vi "Extract positional data on selected miniscan.vi"(8 "error in (no error)":errorcluster, 9 "Display State In":T1={"Numeric"=0.0, "Timeline Ref"=refnum, "Waveform Ref"=refnum, "Fill Plots"=FALSE, "Cursor Redraw"=TRUE}, 11 "Data In":T4) -> (0 "error out":errorcluster, 1 "Extracted intensity data at selected mini-scan location":sgl[](graph))   [LabVIEW 2017, in "XGrapher.xctl"]
uses:
  XGrapher.xctl
  Data 1.ctl
  Typedefs/Xctrl-Data array.ctl
  Typedefs/Xcrtl-Data format definition.ctl
  Typedefs/Xctl-XY data type definition.ctl
  Typedefs/Xctrl-ROI type enum.ctl
  State 1.ctl
  Typedefs/Xctrl-Timeline graph ref.ctl
  Typedefs/Xctrl-Waveform graph ref.ctl
  <userlib>/_OpenG.lib/array/array.llb/Index 1D Array Elements (SGL)__ogtk.vi
panel:
  out "Number of cycles":i32
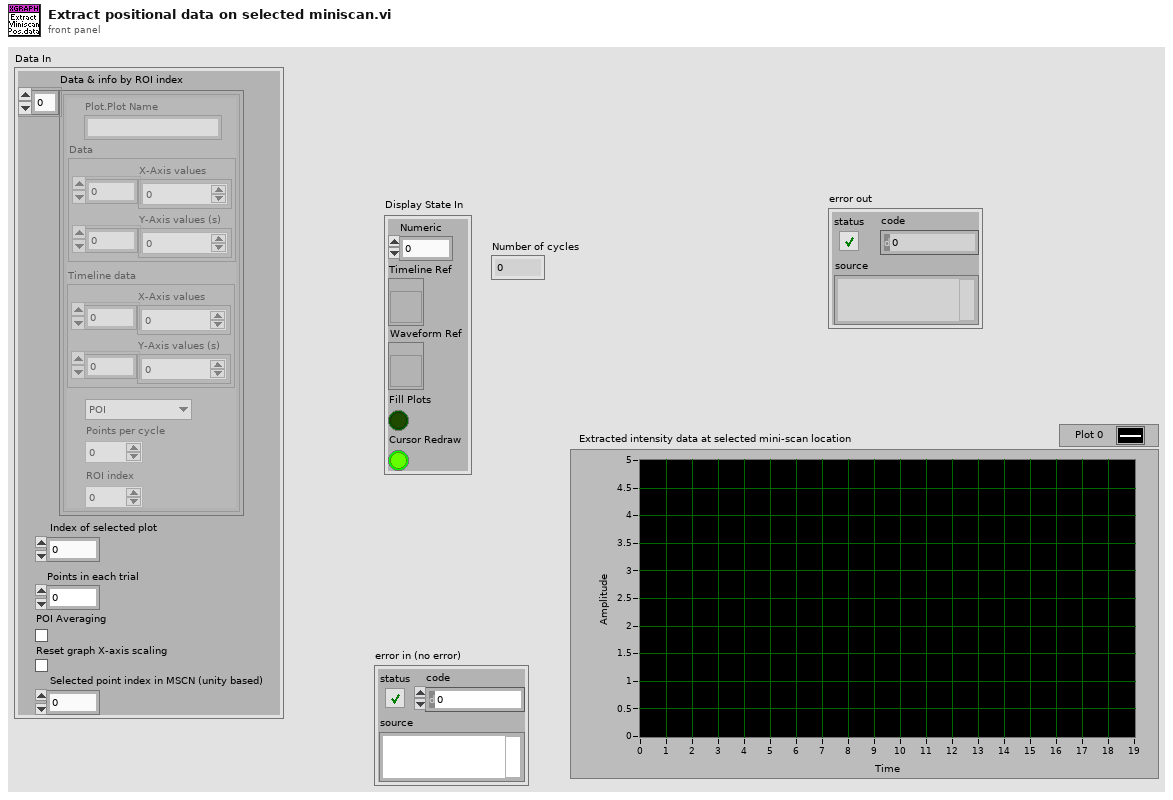
[diagram p1: front panel]
types:
  T1 = typedef "XGrapher.xctl/State 1.ctl" = cluster{"Numeric":dbl, "Timeline Ref":T2, "Waveform Ref":T3, "Fill Plots":bool, "Cursor Redraw":bool}
  T2 = typedef "XGrapher.xctl/Xctrl-Timeline graph ref.ctl" = refnum<vi>
  T3 = typedef "XGrapher.xctl/Xctrl-Waveform graph ref.ctl" = refnum<vi>
  T4 = typedef "XGrapher.xctl/Data 1.ctl" = cluster{"Data & info by ROI index":T5, "Index of selected plot":u16, "Points in each trial":i32, "POI Averaging":bool, "Reset graph X-axis scaling":bool, "Selected point index in MSCN (unity based)":u16}
  T5 = typedef "Xctrl-Data array.ctl" = T6[]
  T6 = typedef "XGrapher.xctl/Xcrtl-Data format definition.ctl" = cluster{"Plot.Plot Name":string, "Data":T7, "Timeline data":T7, "Type":T8, "Points per cycle":u16, "ROI index":u16}
  T7 = typedef "XGrapher.xctl/Xctl-XY data type definition.ctl" = cluster{"X-Axis values":sgl[], "Y-Axis values (s)":sgl[]}
  T8 = typedef "Xctrl-ROI type enum.ctl" = enum16{"POI", "Mini-scan", "Group"}
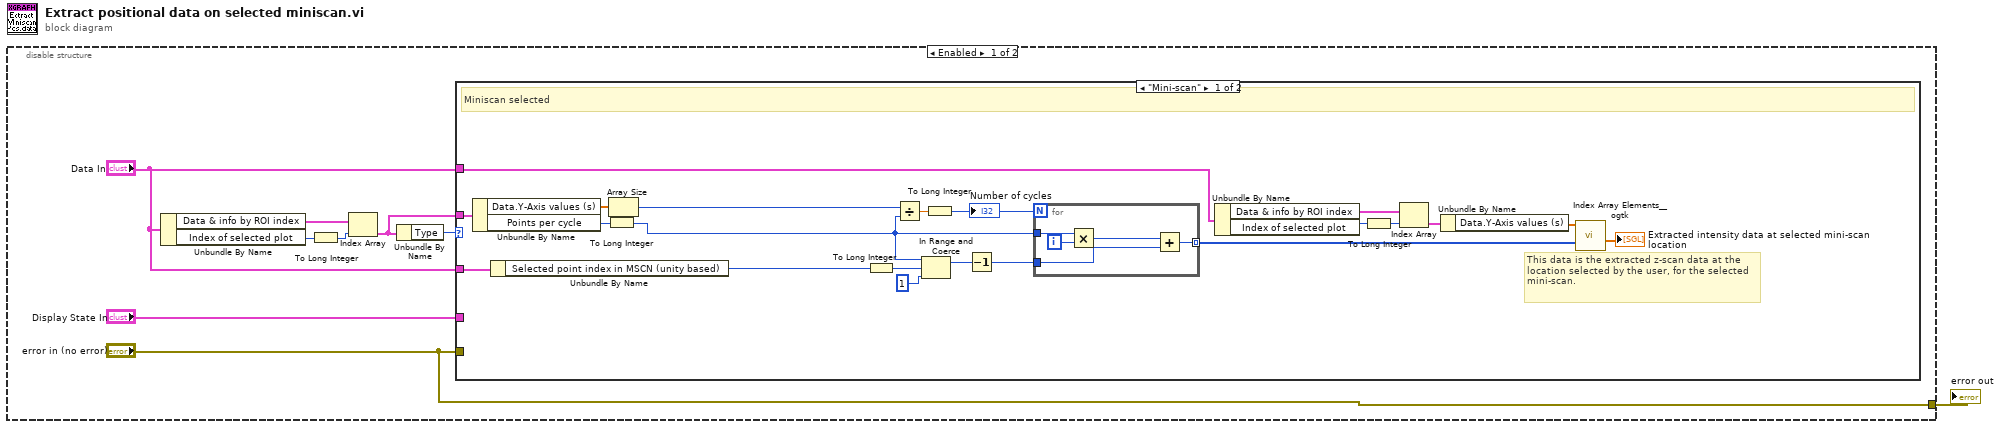
[diagram p0: block diagram]
diagram:
  n1 = disable-structure shown="Enabled" {
    disable-tunnel: ["error in (no error)" _] -> w1
    frame Enabled {
      n2 = Unbundle By Name("Data In") -> ("Data & info by ROI index"=w7:T5, "Index of selected plot"=w8:u16)
      n3 = To Long Integer(number=w8) -> (32bit integer=w6:i32)
      n4 = Index Array(array=w7, index=w6) -> (element=w4:T6)
      n5 = Unbundle By Name(w4) -> ("Type"=w5:T8)
      n6 = case shown="\"Mini-scan\"" w5 {
        tunnel: "Data In" -> [w18 _]
        tunnel: "Display State In" -> [_ _]
        tunnel: "error in (no error)" -> [_ _]
        tunnel: w4 -> [w19 _]
        tunnel: "Data In" -> [w16 _]
        frame "Mini-scan" {
          # "This data is the extracted z-scan data at the location selected by the user, for the selected mini-scan."
          # "Miniscan selected"
          n7 = Unbundle By Name(w19) -> ("Data.Y-Axis values (s)"=w24:sgl[], "Points per cycle"=w15:u16)
          n8 = Unbundle By Name(w16) -> ("Selected point index in MSCN (unity based)"=w17:u16)
          n9 = To Long Integer(number=w15) -> (32bit integer=w13:i32)
          n10 = Array Size(array=w24) -> (size(s)=w27:i32)
          n11 = To Long Integer(number=w17) -> (32bit integer=w10:i32)
          n12 = Divide(x=w27, y=w13) -> (x/y=w26:dbl)
          n13 = In Range and Coerce(upper limit=w13, x=w10, lower limit=1) -> (coerced(x)=w12:i32)  [unwired: 1 out]
          n14 = To Long Integer(number=w26) -> (32bit integer=w25:i32)
          "Number of cycles" <- w25
          n15 = Decrement(x=w12) -> (x-1=w11:i32)
          n16 = for {
            N: w25 -> [_]
            tunnel: [w32] -> w23 mode=indexing
            tunnel: w13 -> [w34]
            tunnel: w11 -> [w31]
            i -> [w35]
            n17 = Multiply(x=w34, y=w35) -> (x*y=w33:i32)
            n18 = Add(x=w33, y=w31) -> (x+y=w32:i32)
          }
          n19 = Unbundle By Name(w18) -> ("Data & info by ROI index"=w29:T5, "Index of selected plot"=w30:u16)
          n20 = To Long Integer(number=w30) -> (32bit integer=w28:i32)
          n21 = Index Array(array=w29, index=w28) -> (element=w22:T6)
          n22 = Unbundle By Name(w22) -> ("Data.Y-Axis values (s)"=w21:sgl[])
          n23 = call-poly <userlib>:"Index Array Elements__ogtk.vi"("indices"=w23, "array"=w21) -> ("elements"=→"Extracted intensity data at selected mini-scan location":sgl[])  [unwired: 9 in]
        }
        frame Default {
          # "Not a miniscan"
        }
      }
    }
    frame Disabled {
    }
  }
  "error out" <- w1
